vi "Cache Files Into Redis.vi"() -> ()   [LabVIEW 2019, in "HTTP Server.lvlib"]
uses:
  HTTP Server.lvlib
  REDIS/Palette/Redis Commands/Connection/AUTH.vi
  REDIS/Palette/Redis Commands/Connection/SELECT.vi
  REDIS/Palette/Redis Commands/Hashes/HSET.vi
panel:
  out "error out":errorcluster
  out "error out 2":errorcluster
  in  "文件根路径":path
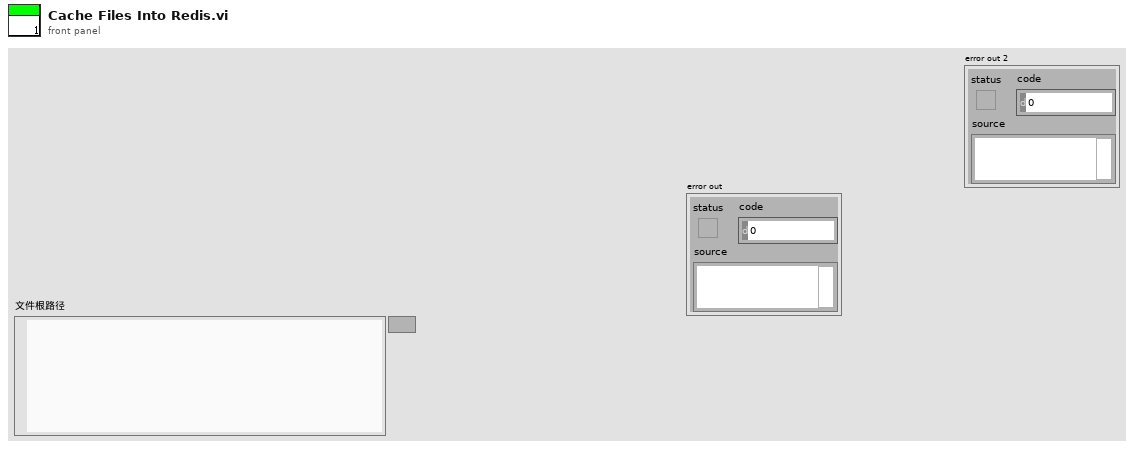
[diagram p1: front panel]
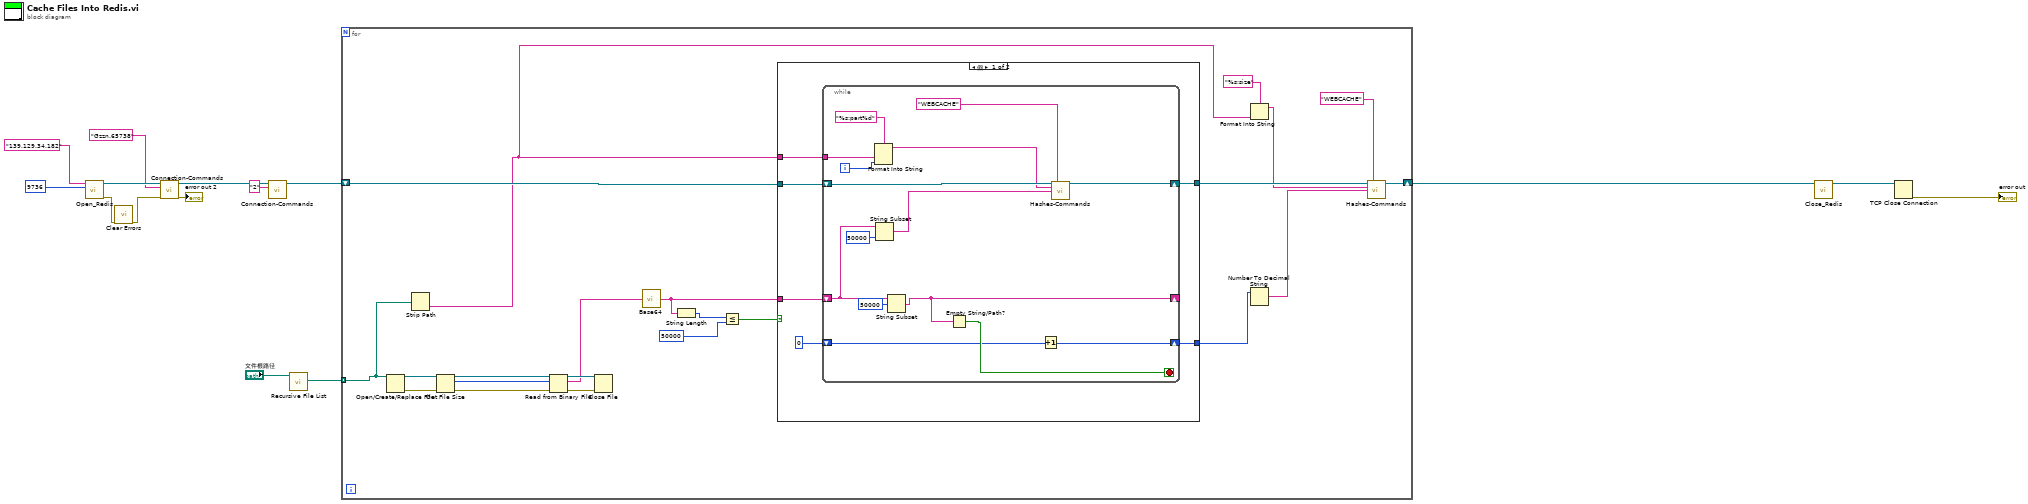
[diagram p0: block diagram]
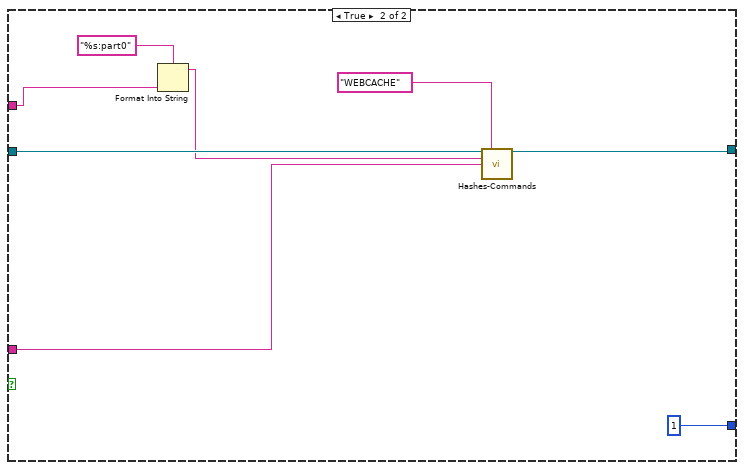
[diagram p2: hidden frame]
diagram:
  n1 = call "Open_Redis.vi"("Host"="139.129.34.182", "Port"=u16 9736) -> ("redis连接ID"=w13:refnum<k5>, "error out"=w8:errorcluster)  [unwired: 11 in, 1 out]
  n2 = call <vilib>:"Clear Errors.vi"("error in (no error)"=w8) -> ("error out"=w7:errorcluster)  [unwired: 5 in, 1 out]
  n3 = call-poly "Connection-Commands.vi"("redis连接ID"=w13, "字符串"="Gzzn.65738", "error in"=w7) -> ("redis连接ID"=w11:refnum<k5>, "error out"=→"error out 2":errorcluster)  [unwired: 10 in, 1 out]
  n4 = call-poly "Connection-Commands.vi"("redis连接ID"=w11, "index"="2") -> ("redis连接ID"=w10:refnum<k5>)  [unwired: 11 in, 2 out]
  n5 = call <vilib>:"Recursive File List.vi"("Folder Path"="文件根路径") -> ("All Files in Dir"=w1:path[])  [unwired: 6 in, 4 out]
  n6 = for {
    shift-right: [w27] -> w3
    shift-left: w10 -> [w37]
    tunnel: w1 -> [w23] mode=indexing
    n7 = Open/Create/Replace File(file path (use dialog)=w23) -> (refnum out=w36:refnum<file>, error out=w35:errorcluster)  [unwired: 5 in, 1 out]
    n8 = Strip Path(path=w23) -> (name=w21:string)  [unwired: 1 out]
    n9 = Get File Size(file=w36, error in=w35) -> (refnum out=w34:refnum<file>, size (in bytes)=w33:i64, 0:w32:errorcluster)
    n10 = Read from Binary File(8:w32, 10:w33, 11:w34) -> (0:w30:errorcluster, 2:w29:string, 3:w31:refnum<file>)  [unwired: 3 in, 1 out]
    n11 = Close File(refnum=w31, error in=w30) -> ()  [unwired: 2 out]
    n12 = call "Base64.vi"("Input String"=w29) -> ("Output String"=w19:string)  [unwired: 6 in]
    n13 = String Length(string=w19) -> (length=w18:i32)
    n14 = Less Or Equal?(x=w18, y=50000) -> (x <= y?=w16:bool)
    n15 = case shown="假" w16 {
      tunnel: w37 -> [w43 w66]
      tunnel: w19 -> [w42 w59]
      tunnel: [w40 w65] -> w28
      tunnel: [w39 1] -> w25
      tunnel: w21 -> [w38 w63]
      frame False {
        n16 = while {
          shift-right: [w58] -> w40
          shift-left: w43 -> [w57]
          shift-right: [w49] -> _
          shift-left: w42 -> [w51]
          shift-right: [w46] -> w39
          shift-left: 0 -> [w47]
          tunnel: w38 -> [w44]
          i -> [w45]
          stop <- w48 stop-if-true
          n17 = Format Into String(format string="%s:part%d" ("Key"), w44, w45) -> (resulting string=w54:string)  [unwired: 2 in, 1 out]
          n18 = String Subset(string=w51, length (rest)=50000 ("长度（剩余）")) -> (substring=w52:string)  [unwired: 1 in]
          n19 = String Subset(string=w51, offset (0)=50000 ("偏移量(0)")) -> (substring=w49:string)  [unwired: 1 in]
          n20 = Empty String/Path?(string/path=w49) -> (empty?=w48:bool)
          n21 = Increment(x=w47) -> (x+1=w46:i32)
          n22 = call-poly "Hashes-Commands.vi"("redis连接ID"=w57, "Key"="WEBCACHE" ("Field"), "Field"=w54, "Value"=w52) -> ("redis连接ID"=w58:refnum<k5>)  [unwired: 9 in, 2 out]
        }
      }
      frame True {
        n23 = Format Into String(format string="%s:part0" ("Key"), w63) -> (resulting string=w61:string)  [unwired: 2 in, 1 out]
        n24 = call-poly "Hashes-Commands.vi"("redis连接ID"=w66, "Key"="WEBCACHE" ("Field"), "Field"=w61, "Value"=w59) -> ("redis连接ID"=w65:refnum<k5>)  [unwired: 9 in, 2 out]
      }
    }
    n25 = Format Into String(format string="%s:size" ("Field"), w21) -> (resulting string=w20:string)  [unwired: 2 in, 1 out]
    n26 = Number To Decimal String(number=w25) -> (decimal integer string=w24:string)  [unwired: 1 in]
    n27 = call-poly "Hashes-Commands.vi"("redis连接ID"=w28, "Key"="WEBCACHE" ("Field"), "Field"=w20, "Value"=w24) -> ("redis连接ID"=w27:refnum<k5>)  [unwired: 9 in, 2 out]
  }
  n28 = call "Close_Redis.vi"("redis连接ID"=w3) -> ("redis连接ID 2"=w5:refnum<k5>)  [unwired: 11 in, 3 out]
  n29 = TCP Close Connection(connection ID=w5) -> (error out=→"error out":errorcluster)  [unwired: 2 in, 1 out]
